vi "bms_daq_gui.vi"() -> ()   [LabVIEW 2022 SP3]
uses:
  <vilib>/Utility/file.llb/Write Delimited Spreadsheet (string).vi
panel:
  in  "File Path":path
  in  "Start Recording":bool
  out "Sync":bool
  out "Cell Voltage":dbl[][](graph)
  out "Cell Temperature":dbl[][](graph)
  out "Balancing State":dbl[][](graph)
  out "Current Balance":string
  out "Current Temperature":string
  out "Current  Voltage":string
  in  "Stop Recording":bool
  in  "Port":refnum<visa-resource-name>
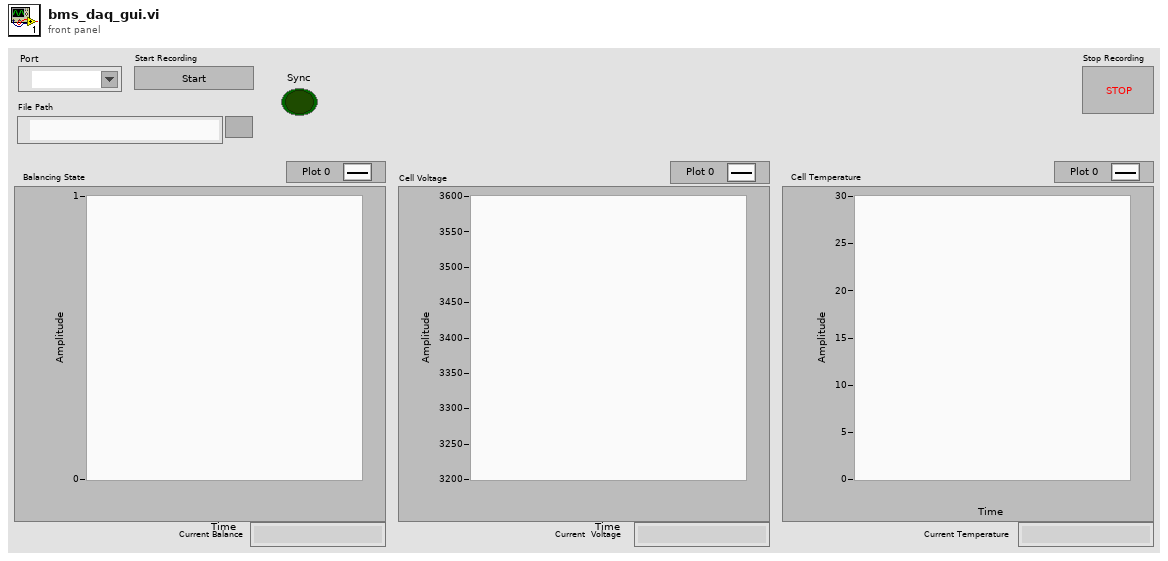
[diagram p1: front panel]
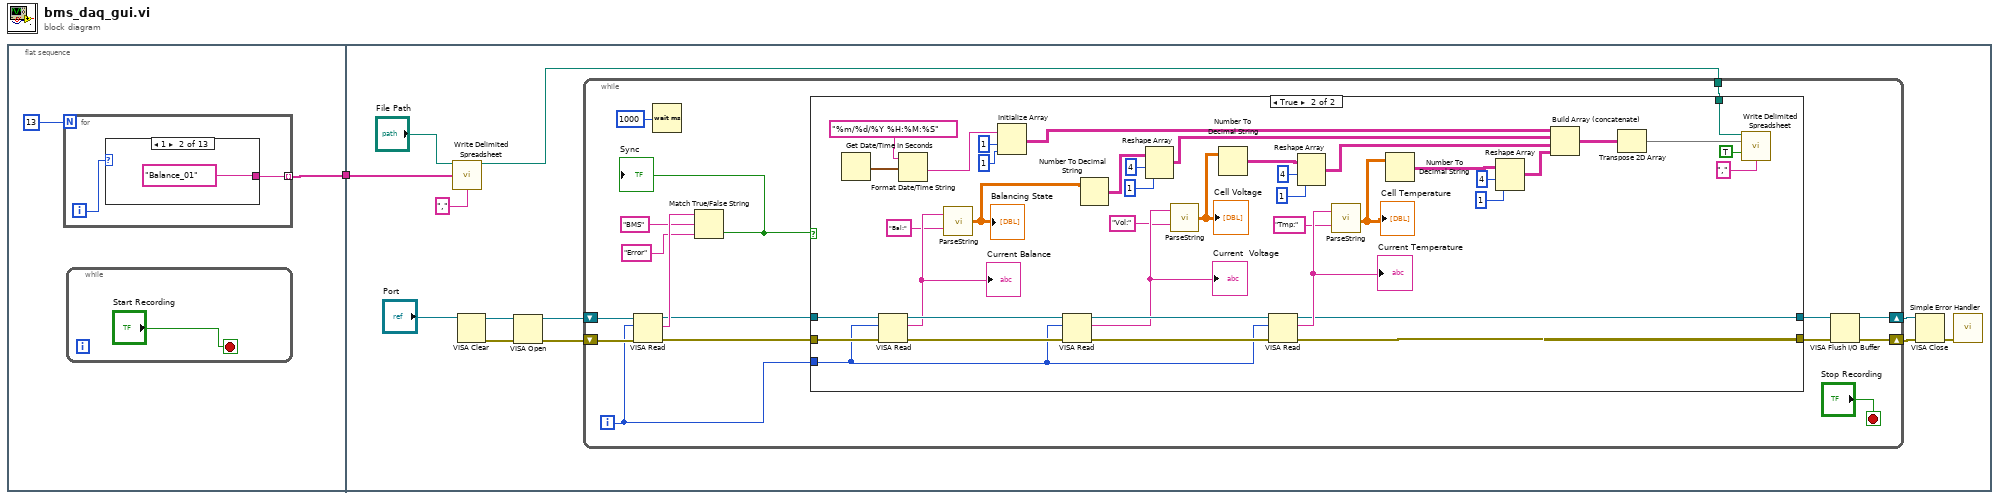
[diagram p0: block diagram]
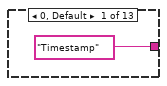
[diagram p2: hidden frame]
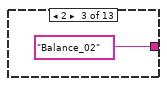
[diagram p3: hidden frame]
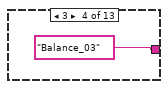
[diagram p4: hidden frame]
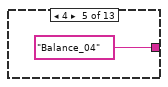
[diagram p5: hidden frame]
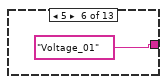
[diagram p6: hidden frame]
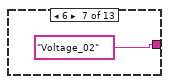
[diagram p7: hidden frame]
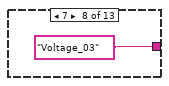
[diagram p8: hidden frame]
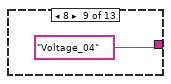
[diagram p9: hidden frame]
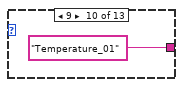
[diagram p10: hidden frame]
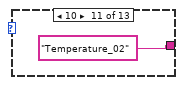
[diagram p11: hidden frame]
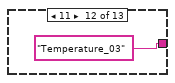
[diagram p12: hidden frame]
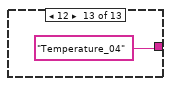
[diagram p13: hidden frame]
diagram:
  n1 = flat-sequence {
    tunnel: [w2] -> w1
    tunnel: w1 -> [w23]
    frame #0 {
      n2 = for {
        N: 13 -> [_]
        tunnel: [w4] -> w2 mode=indexing
        i -> [w5]
        n3 = case shown="1" w5 {
          tunnel: ["Timestamp" "Balance_01" "Balance_02" "Balance_03" "Balance_04" "Voltage_01" "Voltage_02" "Voltage_03" "Voltage_04" "Temperature_01" "Temperature_02" "Temperature_03" "Temperature_04"] -> w4
          frame 0, Default {
          }
          frame 1 {
          }
          frame 2 {
          }
          frame 3 {
          }
          frame 4 {
          }
          frame 5 {
          }
          frame 6 {
          }
          frame 7 {
          }
          frame 8 {
          }
          frame 9 {
          }
          frame 10 {
          }
          frame 11 {
          }
          frame 12 {
          }
        }
      }
      n4 = while {
        stop <- "Start Recording" stop-if-true
      }
    }
    frame #1 {
      n5 = call-poly <vilib>:"Write Delimited Spreadsheet.vi"("file path (dialog if empty)"="File Path", "1D data"=w23, "delimiter (\\t)"="," ("delimiter (\\t)")) -> ("new file path (Not A Path if cancelled)"=w22:path)  [unwired: 11 in, 1 out]
      n6 = VISA Clear(VISA resource name="Port") -> (VISA resource name out=w28:refnum<visa-resource-name>, error out=w29:errorcluster)  [unwired: 1 in]
      n7 = VISA Open(error in (no error)=w29, VISA resource name=w28) -> (VISA resource name=w26:refnum<visa-resource-name>, error out=w27:errorcluster)  [unwired: 3 in]
      n8 = while {
        shift-right: [w38] -> w30
        shift-left: w26 -> [w45]
        shift-right: [w37] -> w25
        shift-left: w27 -> [w44]
        tunnel: w22 -> [w32]
        i -> [w39]
        stop <- "Stop Recording" stop-if-true
        n9 = VISA Read(VISA resource name=w45, byte count=w39, error in (no error)=w44) -> (VISA resource name out=w41:refnum<visa-resource-name>, read buffer=w43:string, error out=w40:errorcluster)  [unwired: 1 out]
        n10 = Wait (ms)(milliseconds to wait=u32 1000) -> ()  [unwired: 1 out]
        n11 = Match True/False String(2:"Error" ("false string"), 3:"BMS" ("true string"), 4:w43) -> (0:w33:bool)  [unwired: 1 out]
        "Sync" <- w33
        n12 = case shown="True" w33 {
          tunnel: w41 -> [w49 w80]
          tunnel: w40 -> [w48 w79]
          tunnel: w39 -> [_ w78]
          tunnel: [w49 w77] -> w36
          tunnel: [w48 w76] -> w35
          tunnel: w32 -> [_ w73]
          frame False {
          }
          frame True {
            n13 = Get Date/Time In Seconds() -> (seconds since 1Jan1904=w75:timestamp)
            n14 = VISA Read(VISA resource name=w80, byte count=w78, error in (no error)=w79) -> (VISA resource name out=w87:refnum<visa-resource-name>, read buffer=w86:string, error out=w90:errorcluster)  [unwired: 1 out]
            "Current Balance" <- w86
            n15 = Format Date/Time String(time format string (%c)="%m/%d/%Y %H:%M:%S", seconds (now)=w75) -> (date/time string=w69:string)  [unwired: 1 in]
            n16 = call "ParseString.vi"("Input String"=w86, "Classifier"="Bal:") -> ("Output Array"=w72:dbl[][])  [unwired: 17 in]
            "Balancing State" <- w72
            n17 = Initialize Array(w69, 1 ("dimension size"), 1 ("dimension size")) -> (w54:string[][])
            n18 = VISA Read(VISA resource name=w87, byte count=w78, error in (no error)=w90) -> (VISA resource name out=w89:refnum<visa-resource-name>, read buffer=w85:string, error out=w88:errorcluster)  [unwired: 1 out]
            "Current  Voltage" <- w85
            n19 = Number To Decimal String(number=w72) -> (decimal integer string=w66:string[][])  [unwired: 1 in]
            n20 = Reshape Array(w66, 4 ("dimension size"), 1 ("dimension size")) -> (w55:string[][])
            n21 = call "ParseString.vi"("Input String"=w85, "Classifier"="Vol:") -> ("Output Array"=w71:dbl[][])  [unwired: 17 in]
            "Cell Voltage" <- w71
            n22 = Number To Decimal String(number=w71) -> (decimal integer string=w59:string[][])  [unwired: 1 in]
            n23 = VISA Read(VISA resource name=w89, byte count=w78, error in (no error)=w88) -> (VISA resource name out=w77:refnum<visa-resource-name>, read buffer=w84:string, error out=w76:errorcluster)  [unwired: 1 out]
            "Current Temperature" <- w84
            n24 = Reshape Array(w59, 4 ("dimension size"), 1 ("dimension size")) -> (w56:string[][])
            n25 = call "ParseString.vi"("Input String"=w84, "Classifier"="Tmp:") -> ("Output Array"=w70:dbl[][])  [unwired: 17 in]
            "Cell Temperature" <- w70
            n26 = Number To Decimal String(number=w70) -> (decimal integer string=w58:string[][])  [unwired: 1 in]
            n27 = Reshape Array(w58, 4 ("dimension size"), 1 ("dimension size")) -> (w57:string[][])
            n28 = Build Array (concatenate)(w54, w55, w56, w57) -> (w51:string[][])
            n29 = Transpose 2D Array(2D array=w51) -> (transposed array=w50:string[][])
            n30 = call-poly <vilib>:"Write Delimited Spreadsheet.vi"("file path (dialog if empty)"=w73, "2D data"=w50, "append to file? (new file:F)"=TRUE, "delimiter (\\t)"="," ("delimiter (\\t)")) -> ()  [unwired: 10 in, 2 out]
          }
        }
        n31 = VISA Flush I/O Buffer(VISA resource name=w36, error in (no error)=w35) -> (VISA resource name out=w38:refnum<visa-resource-name>, error out=w37:errorcluster)  [unwired: 1 in]
      }
      n32 = VISA Close(VISA resource name=w30, error in (no error)=w25) -> (error out=w31:errorcluster)
      n33 = call <vilib>:"Simple Error Handler.vi"("error in (no error)"=w31) -> ()  [unwired: 4 in, 5 out]
    }
  }
